vi "Insert Category.vi"(8 "error in (no error)":errorcluster, 10 "name":string, 11 "Database in":refnum<class "Database.lvclass">) -> (0 "error out":errorcluster, 3 "Database out":refnum<class "Database.lvclass">)   [LabVIEW 2018, in "Database.lvclass"]
uses:
  Database.lvclass
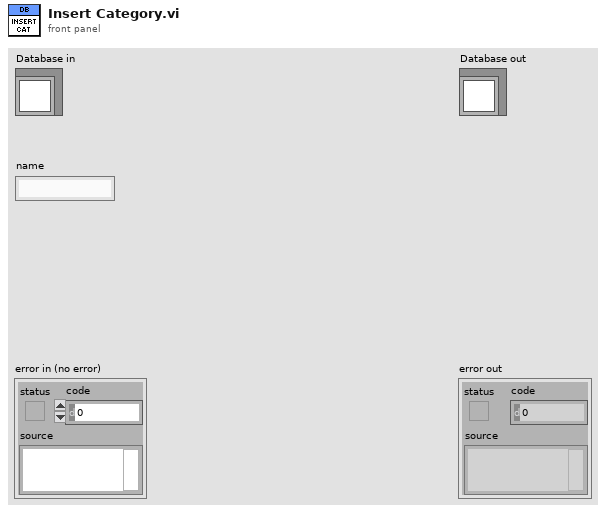
[diagram p1: front panel]
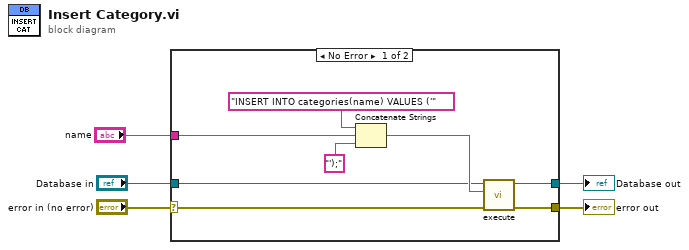
[diagram p0: block diagram]
diagram:
  n1 = case shown="No Error" "error in (no error)" {
    selector: "error in (no error)" -> [w7 w15]
    tunnel: [w8 w15] -> w4
    tunnel: [w9 w14] -> w2
    tunnel: "Database in" -> [w10 w14]
    tunnel: "name" -> [w6 _]
    frame No Error {
      n2 = Concatenate Strings("INSERT INTO categories(name) VALUES ('", w6, "');" ("string")) -> (w11:string)
      n3 = call "execute.vi"("error in (no error)"=w7, "SQL query"=w11, "Database in"=w10) -> ("error out"=w8:errorcluster, "Database out"=w9:refnum<class "Database.lvclass">)  [unwired: 7 in]
    }
    frame Error {
    }
  }
  "error out" <- w4
  "Database out" <- w2
